vi "curva subvão.vi"(8 "error in":errorcluster, 11 "Dados SP":T1={"Condutor"={"Pc (N/m)"=0.0, "Mod.Young (N/m²)"=0.0, "Dil.Term.c (m/°C)"=0.0, "Área  (m²)"=0.0, "Tração EDS (N)"=0.0, "Tração Torig(N)"=0.0, "Tração Talta (N)"=0.0}, "Suporte"={"Ps (N/m)"=0.0, "Es (N/m²)"=0.0, "DTc (1/°C)"=0.0, "Área sup (m²)"=0.0, "Tração EDS sup (N)"=0.0, "Tração AT sup (N)"=0.0, "Flecha sup AT (m)"=0.0}, "Projeto"={"Temp. EDS (°C)"=0.0, "Lim.original (°C)"=0.0, "Lim.extend. (°C)"=0.0, "N. cabo/fase"=1.0}, "Vetor de dados"={"Coor.X.esp"=[], "Coor.Y.Esp."=[], "Sub.vao X"=[], "Sub.vao Y"=[], "CoordY.sup"=[], "CoordX.sup"=[]}, "Subvão"={"N. Esp."=0.0, "F.lim (m)"=0.0, "Ext.calc"=0.0, "Ext.definido"=0.0, "Comp.cabo"=0.0, "Ext.55%"=0.0, "Tração sub\nAT (N)"=0.0, "Ext.sel."=0.0, "Flecha lim.\ncalc (m)"=0.0}, "Vão"={"Extensão (m)"=0.0, "Desnivel (m)"=0.0, "Ext.Lim sub (m)"=0.0, "Flecha à 60 °C"=0.0}} {"Projeto"."N. cabo/fase" min=1.0 max=8.0 step=1.0 format="%#_1f"}) -> (0 "error out":errorcluster, 2 "Subvão esp.":cluster{dbl[], dbl[]}, 3 "Dados SP Out":T1={"Condutor"={"Pc (N/m)"=0.0, "Mod.Young (N/m²)"=0.0, "Dil.Term.c (m/°C)"=0.0, "Área  (m²)"=0.0, "Tração EDS (N)"=0.0, "Tração Torig(N)"=0.0, "Tração Talta (N)"=0.0}, "Suporte"={"Ps (N/m)"=0.0, "Es (N/m²)"=0.0, "DTc (1/°C)"=0.0, "Área sup (m²)"=0.0, "Tração EDS sup (N)"=0.0, "Tração AT sup (N)"=0.0, "Flecha sup AT (m)"=0.0}, "Projeto"={"Temp. EDS (°C)"=0.0, "Lim.original (°C)"=0.0, "Lim.extend. (°C)"=0.0, "N. cabo/fase"=1.0}, "Vetor de dados"={"Coor.X.esp"=[], "Coor.Y.Esp."=[], "Sub.vao X"=[], "Sub.vao Y"=[], "CoordY.sup"=[], "CoordX.sup"=[]}, "Subvão"={"N. Esp."=0.0, "F.lim (m)"=0.0, "Ext.calc"=0.0, "Ext.definido"=0.0, "Comp.cabo"=0.0, "Ext.55%"=0.0, "Tração sub\nAT (N)"=0.0, "Ext.sel."=0.0, "Flecha lim.\ncalc (m)"=0.0}, "Vão"={"Extensão (m)"=0.0, "Desnivel (m)"=0.0, "Ext.Lim sub (m)"=0.0, "Flecha à 60 °C"=0.0}} {"Projeto"."N. cabo/fase" min=1.0 max=8.0 step=1.0 format="%#_1f"})   [LabVIEW 2020]
uses:
  controles/SP data.ctl
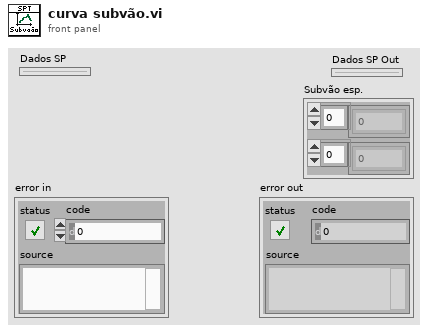
[diagram p1: front panel]
types:
  T1 = typedef "SP data.ctl" = cluster{"Condutor":cluster{"Pc (N/m)":dbl, "Mod.Young (N/m²)":dbl, "Dil.Term.c (m/°C)":dbl, "Área  (m²)":dbl, "Tração EDS (N)":dbl, "Tração Torig(N)":dbl, "Tração Talta (N)":dbl}, "Suporte":cluster{"Ps (N/m)":dbl, "Es (N/m²)":dbl, "DTc (1/°C)":dbl, "Área sup (m²)":dbl, "Tração EDS sup (N)":dbl, "Tração AT sup (N)":dbl, "Flecha sup AT (m)":dbl}, "Projeto":cluster{"Temp. EDS (°C)":dbl, "Lim.original (°C)":dbl, "Lim.extend. (°C)":dbl, "N. cabo/fase":dbl}, "Vetor de dados":cluster{"Coor.X.esp":dbl[], "Coor.Y.Esp.":dbl[], "Sub.vao X":dbl[], "Sub.vao Y":dbl[], "CoordY.sup":dbl[], "CoordX.sup":dbl[]}, "Subvão":cluster{"N. Esp.":dbl, "F.lim (m)":dbl, "Ext.calc":dbl, "Ext.definido":dbl, "Comp.cabo":dbl, "Ext.55%":dbl, "Tração sub\nAT (N)":dbl, "Ext.sel.":dbl, "Flecha lim.\ncalc (m)":dbl}, "Vão":cluster{"Extensão (m)":dbl, "Desnivel (m)":dbl, "Ext.Lim sub (m)":dbl, "Flecha à 60 °C":dbl}}
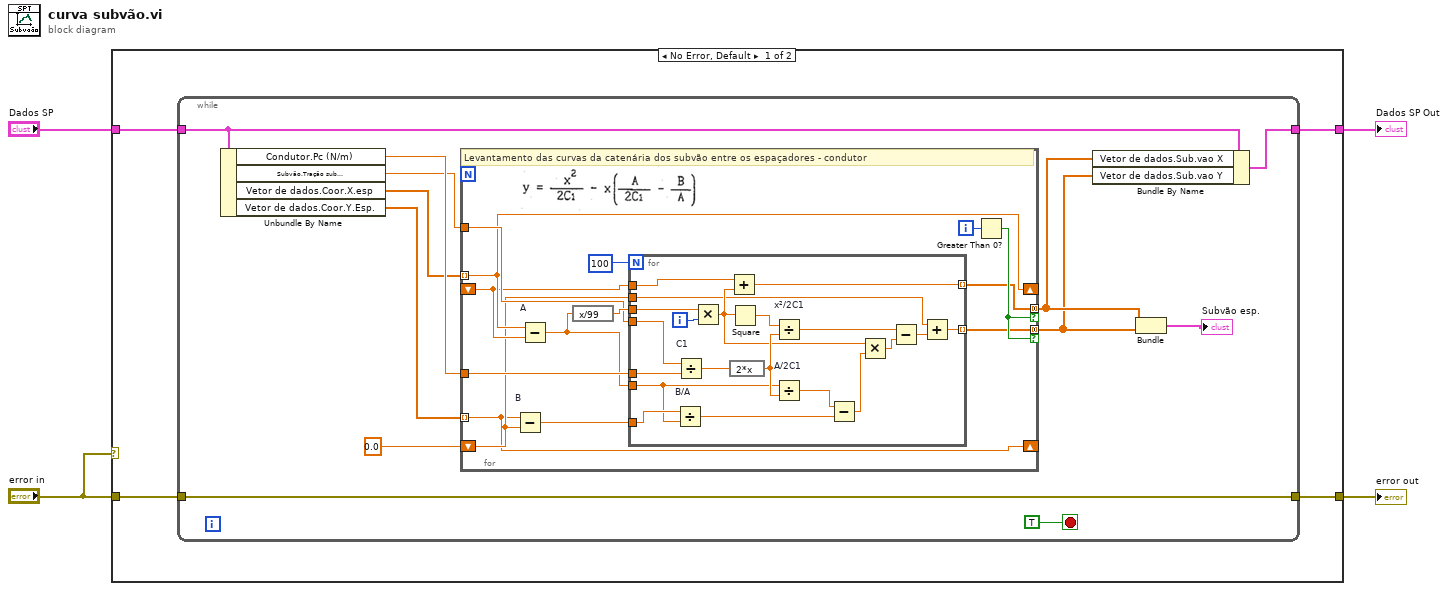
[diagram p0: block diagram]
diagram:
  n1 = case shown="No Error, Default" "error in" {
    tunnel: "Dados SP" -> [w8 w56]
    tunnel: "error in" -> [w7 w55]
    tunnel: [w6 w55] -> w3
    tunnel: [w5 w56] -> w2
    frame No Error {
      n2 = while {
        tunnel: w8 -> [w15]
        tunnel: w7 -> [w17]
        tunnel: [w17] -> w6
        tunnel: [w14] -> w5
        stop <- TRUE stop-if-true
        n3 = Unbundle By Name(w15) -> ("Condutor.Pc (N/m)"=w19:dbl, "Subvão.Tração sub\nAT (N)"=w16:dbl, "Vetor de dados.Coor.X.esp"=w13:dbl[], "Vetor de dados.Coor.Y.Esp."=w12:dbl[])
        n4 = for {
          tunnel: w12 -> [w21] mode=indexing
          shift-right: [w21] -> _
          shift-left: 0.0 -> [w22]
          tunnel: [w24] -> w11 mode=concatenating if=w27
          tunnel: w13 -> [w26] mode=indexing
          shift-right: [w26] -> _
          shift-left: _ -> [w25]
          tunnel: w19 -> [w32]
          tunnel: w16 -> [w28]
          tunnel: [w23] -> w10 mode=concatenating if=w27
          i -> [w34]
          # "Levantamento das curvas da catenária dos subvão entre os espaçadores - condutor"
          n5 = Subtract "B"(x=w21, y=w22) -> (x-y=w33:dbl)
          n6 = Subtract "A"(x=w26, y=w25) -> (x-y=w30:dbl)
          n7 = expression code="x/99"(w30) -> (w29:dbl)
          n8 = for {
            N: 100 -> [_]
            tunnel: w33 -> [w46]
            tunnel: w30 -> [w35]
            tunnel: w32 -> [w45]
            tunnel: w29 -> [w44]
            tunnel: [w41] -> w24 mode=indexing
            tunnel: [w38] -> w23 mode=indexing
            tunnel: w28 -> [w42]
            tunnel: w25 -> [w39]
            tunnel: w22 -> [w36]
            i -> [w43]
            n9 = Divide "B/A"(x=w46, y=w35) -> (x/y=w52:dbl)
            n10 = Divide "C1"(x=w42, y=w45) -> (x/y=w54:dbl)
            n11 = Multiply(x=w44, y=w43) -> (x*y=w40:dbl)
            n12 = Add(x=w39, y=w40) -> (x+y=w41:dbl)
            n13 = Square(x=w40) -> (x^2=w48:dbl)
            n14 = expression code="2*x"(w54) -> (w49:dbl)
            n15 = Divide "x²/2C1"(x=w48, y=w49) -> (x/y=w47:dbl)
            n16 = Divide "A/2C1"(x=w35, y=w49) -> (x/y=w53:dbl)
            n17 = Subtract(x=w53, y=w52) -> (x-y=w51:dbl)
            n18 = Multiply(x=w40, y=w51) -> (x*y=w50:dbl)
            n19 = Subtract(x=w47, y=w50) -> (x-y=w37:dbl)
            n20 = Add(x=w36, y=w37) -> (x+y=w38:dbl)
          }
          n21 = Greater Than 0?(x=w34) -> (x > 0?=w27:bool)
        }
        n22 = Bundle By Name(cluster=w15, "Vetor de dados.Sub.vao X"=w11, "Vetor de dados.Sub.vao Y"=w10) -> (w14:T1)
        n23 = Bundle(w11, w10) -> (→"Subvão esp.":cluster{dbl[], dbl[]})  [unwired: 1 in]
      }
    }
    frame Error {
    }
  }
  "Dados SP Out" <- w2
  "error out" <- w3
